vi "Listbox-Toggle Checked Item.vi"(8 "error in (no error)":errorcluster, 9 "index":i32, 11 "reference":refnum<vi>) -> (0 "error out":errorcluster, 1 "checked?":bool, 3 "reference out":refnum<vi>)   [LabVIEW 2020]
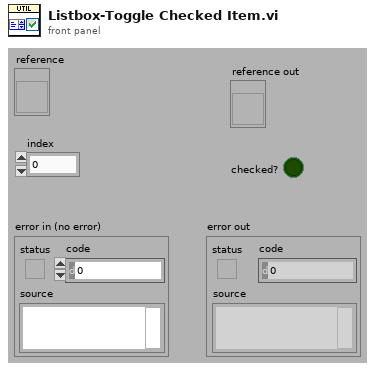
[diagram p1: front panel]
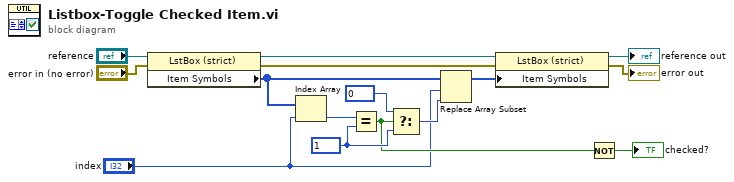
[diagram p0: block diagram]
diagram:
  w13 = 1
  n1 = property on="Property Node" class="LstBox (strict)"(reference="reference", error in="error in (no error)") -> (reference out=w3:refnum<vi>, error out=w2:errorcluster, "Item Symbols"=w10:i32[])
  n2 = Index Array(array=w10, index="index") -> (element=w11:i32)
  n3 = Equal?(x=w11, y=w13) -> (x = y?=w12:bool)
  n4 = Select(t=0, s=w12, f=w13) -> (s? t:f=w15:i32)
  n5 = Replace Array Subset(array=w10, new element=w15, index="index") -> (w9:i32[])
  n6 = property on="Property Node" class="LstBox (strict)"(reference=w3, error in=w2, "Item Symbols"=w9) -> (reference out=→"reference out":refnum<vi>, error out=→"error out":errorcluster)
  n7 = Not(x=w12) -> (.not. x?=→"checked?":bool)
